vi "Clear Annotation.vi"(8 "error in (no error)":errorcluster, 11 "FSM.Edge in":refnum<class "FSM.Edge.lvclass">) -> (0 "error out":errorcluster, 3 "FSM.Edge out":refnum<class "FSM.Edge.lvclass">)   [LabVIEW 2015, in "FSM.Edge.lvclass"]
uses:
  FSM.Edge.lvclass
  FSM.Edge.lvclass/FSM.Edge.ctl
  FSM.Annotation/FSM.Annotation.lvclass
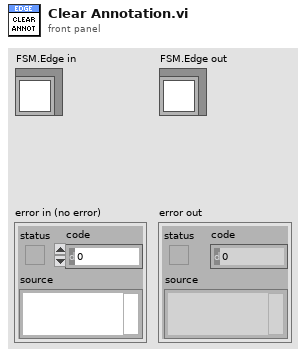
[diagram p1: front panel]
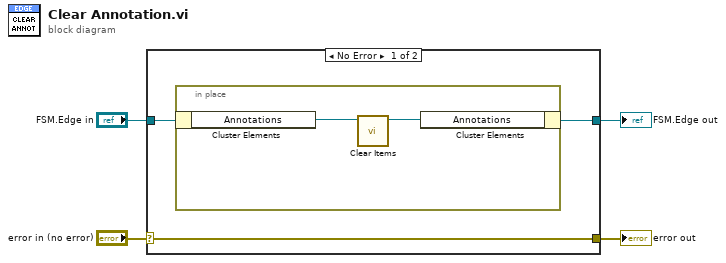
[diagram p0: block diagram]
diagram:
  n1 = case shown="No Error" "error in (no error)" {
    selector: "error in (no error)" -> [w7 w11]
    tunnel: [w7 w11] -> w3
    tunnel: [w5 w10] -> w2
    tunnel: "FSM.Edge in" -> [w6 w10]
    frame No Error {
      n2 = in-place {
        n3 = in-place-cluster #1(w6) -> ("Annotations"=w9:refnum<class "FSM.Annotation.lvclass">)
        n4 = call "Clear Items.vi"("FSM.Annotation in"=w9) -> ("FSM.Annotation out"=w8:refnum<class "FSM.Annotation.lvclass">)  [unwired: 9 in, 1 out]
        n5 = in-place-cluster #1("Annotations"=w8) -> (w5:refnum<class "FSM.Edge.lvclass">)
      }
    }
    frame Error {
    }
  }
  "error out" <- w3
  "FSM.Edge out" <- w2
